vi "prep_plotting_data.vi"(2 "Plotting Data":T2) -> (5 "C1 (time)":T1, 6 "C2 (time)":T1, 7 "C1 (mass)":cluster{dbl, cluster{dbl[], "Y":dbl[]}}, 8 "C2 (mass)":cluster{dbl, cluster{dbl[], "Y":dbl[]}})   [LabVIEW 2023]
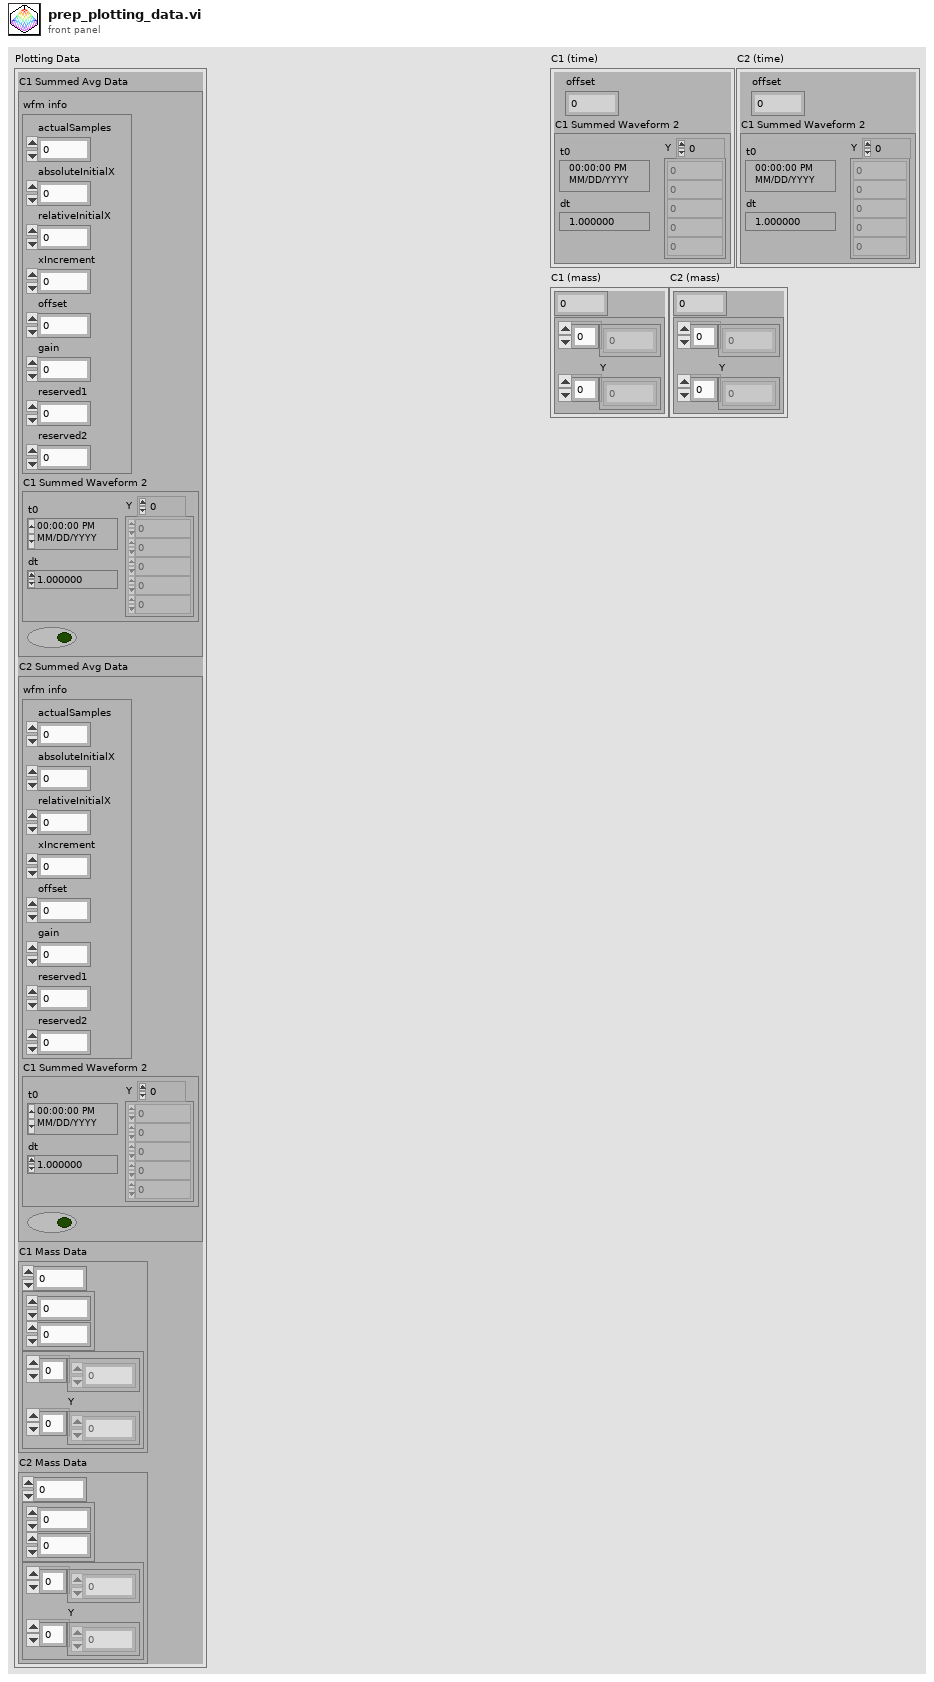
[diagram p1: front panel]
types:
  T1 = cluster{"offset":dbl, "C1 Summed Waveform 2":waveform(dbl)}
  T2 = cluster{"C1 Summed Avg Data":cluster{"wfm info":cluster{"actualSamples":i32, "absoluteInitialX":dbl, "relativeInitialX":dbl, "xIncrement":dbl, "offset":dbl, "gain":dbl, "reserved1":dbl, "reserved2":dbl}, "C1 Summed Waveform 2":waveform(dbl), bool}, "C2 Summed Avg Data":cluster{"wfm info":cluster{"actualSamples":i32, "absoluteInitialX":dbl, "relativeInitialX":dbl, "xIncrement":dbl, "offset":dbl, "gain":dbl, "reserved1":dbl, "reserved2":dbl}, "C1 Summed Waveform 2":waveform(dbl), bool}, "C1 Mass Data":cluster{dbl, cluster{dbl, dbl}, cluster{dbl[], "Y":dbl[]}}, "C2 Mass Data":cluster{dbl, cluster{dbl, dbl}, cluster{dbl[], "Y":dbl[]}}}
  T3 = cluster{"wfm info":cluster{"actualSamples":i32, "absoluteInitialX":dbl, "relativeInitialX":dbl, "xIncrement":dbl, "offset":dbl, "gain":dbl, "reserved1":dbl, "reserved2":dbl}, "C1 Summed Waveform 2":waveform(dbl), bool}
  T4 = cluster{dbl, cluster{dbl, dbl}, cluster{dbl[], "Y":dbl[]}}
  T5 = cluster{"actualSamples":i32, "absoluteInitialX":dbl, "relativeInitialX":dbl, "xIncrement":dbl, "offset":dbl, "gain":dbl, "reserved1":dbl, "reserved2":dbl}
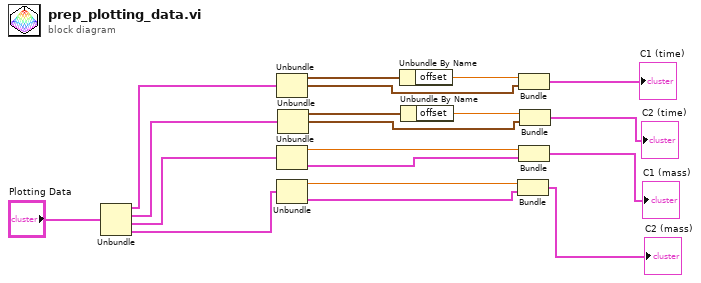
[diagram p0: block diagram]
diagram:
  n1 = Unbundle("Plotting Data") -> ("C1 Summed Avg Data"=w18:T3, "C2 Summed Avg Data"=w11:T3, "C1 Mass Data"=w10:T4, "C2 Mass Data"=w9:T4)
  n2 = Unbundle(w18) -> ("wfm info"=w17:T5, "C1 Summed Waveform 2"=w15:waveform(dbl))  [unwired: 1 out]
  n3 = Unbundle(w10) -> (w7:dbl, w8:cluster{dbl[], "Y":dbl[]})  [unwired: 1 out]
  n4 = Unbundle(w9) -> (w6:dbl, w5:cluster{dbl[], "Y":dbl[]})  [unwired: 1 out]
  n5 = Unbundle(w11) -> ("wfm info"=w14:T5, "C1 Summed Waveform 2"=w12:waveform(dbl))  [unwired: 1 out]
  n6 = Unbundle By Name(w17) -> ("offset"=w16:dbl)
  n7 = Unbundle By Name(w14) -> ("offset"=w13:dbl)
  n8 = Bundle(w6, w5) -> (→"C2 (mass)":cluster{dbl, cluster{dbl[], "Y":dbl[]}})  [unwired: 1 in]
  n9 = Bundle("offset"=w16, "C1 Summed Waveform 2"=w15) -> (→"C1 (time)":T1)  [unwired: 1 in]
  n10 = Bundle(w7, w8) -> (→"C1 (mass)":cluster{dbl, cluster{dbl[], "Y":dbl[]}})  [unwired: 1 in]
  n11 = Bundle("offset"=w13, "C1 Summed Waveform 2"=w12) -> (→"C2 (time)":T1)  [unwired: 1 in]
